vi "Count Update.vi"(8 "error in":errorcluster, 11 "OutputClusterIn":T1={"Acknowledgement"={"Enqueuer"=refnum, "VIReference"=refnum, "VIName"=""}, "AllPartInfo"=[{"PartName"="", "NumberOfRacks"=0, "MeasurementIDsArray"=[], "MeasurementNamesArray"=[], "SpecValuesArray"=[]}], "PartInfo"={"PartName"="", "TotalCount"=0, "ReelCount"=0, "NumberOfRacks"=0, "MeasurementIDsArray"=[], "MeasurementNamesArray"=[], "SpecValuesArray"=[]}, "Result Cluster"={"Measurement Names Array"=[], "Pass-Fail Array"=[], "Measurement Values Array "=[], "Roi for overlay (Arrows) Array"=[], "Algo Type Array"=[], "Image Array"=[], "Clamp operations"=enum."Average Clamp", "  Search Direction "=[], "Images_Array_in"=[], "ResultPF"=FALSE, "Total Cluster Values"={"Total Fail"=0, "Total Pass"=0, "Total Count"=0}, "Reel Counter Cluster"={"Reel Fail"=0, "Reel Pass"=0, "Reel Count"=0}, "Tolerance  Array"=[], "Array of Cam Spec Control Bool"=[], "Control Pass Fail Array"=[], "Specification Pass Fail Array"=[], "Overlay Arrow Lines"=[], "Camera ID"=[], "Trigger count"=0, "Specification fail?"=FALSE}, "ErrorMessage"=""}) -> (0 "error out":errorcluster, 3 "OutputClusterOut":T1={"Acknowledgement"={"Enqueuer"=refnum, "VIReference"=refnum, "VIName"=""}, "AllPartInfo"=[{"PartName"="", "NumberOfRacks"=0, "MeasurementIDsArray"=[], "MeasurementNamesArray"=[], "SpecValuesArray"=[]}], "PartInfo"={"PartName"="", "TotalCount"=0, "ReelCount"=0, "NumberOfRacks"=0, "MeasurementIDsArray"=[], "MeasurementNamesArray"=[], "SpecValuesArray"=[]}, "Result Cluster"={"Measurement Names Array"=[], "Pass-Fail Array"=[], "Measurement Values Array "=[], "Roi for overlay (Arrows) Array"=[], "Algo Type Array"=[], "Image Array"=[], "Clamp operations"=enum."Average Clamp", "  Search Direction "=[], "Images_Array_in"=[], "ResultPF"=FALSE, "Total Cluster Values"={"Total Fail"=0, "Total Pass"=0, "Total Count"=0}, "Reel Counter Cluster"={"Reel Fail"=0, "Reel Pass"=0, "Reel Count"=0}, "Tolerance  Array"=[], "Array of Cam Spec Control Bool"=[], "Control Pass Fail Array"=[], "Specification Pass Fail Array"=[], "Overlay Arrow Lines"=[], "Camera ID"=[], "Trigger count"=0, "Specification fail?"=FALSE}, "ErrorMessage"=""})   [LabVIEW 2019, in "Algorithm.lvclass"]
uses:
  FrameworkOverrides/Algorithm.lvclass
  Controls/OutputCluster.ctl
  Common/Controls/AllPartInfo.ctl
  Common/Controls/Acknowledgement.ctl
  <vilib>/ActorFramework/Message Enqueuer/Message Enqueuer.lvclass
  Controls/Result Cluster.ctl
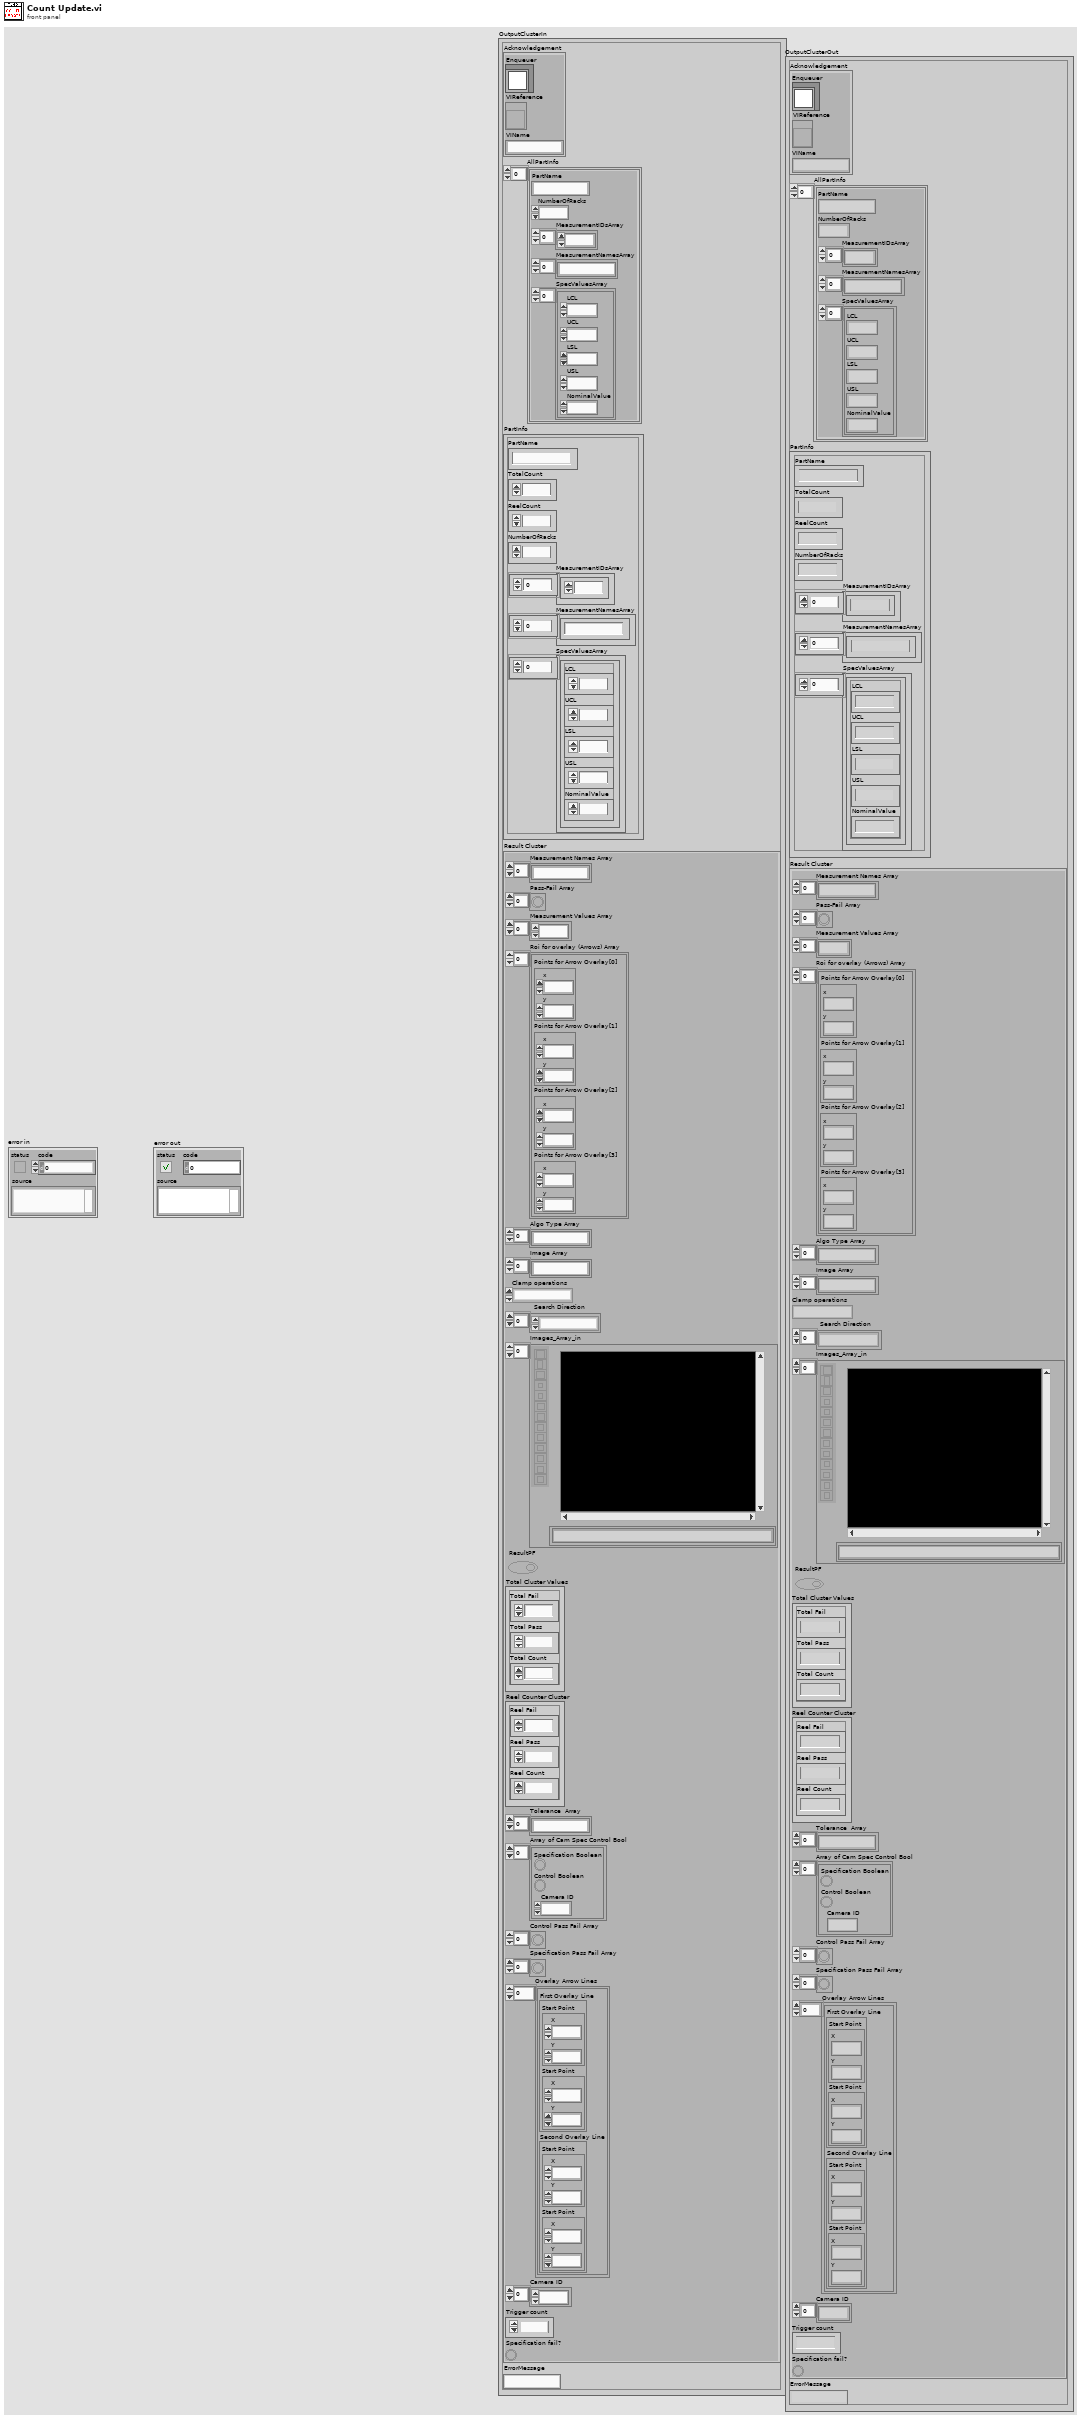
[diagram p1: front panel]
types:
  T1 = typedef "Algorithm.lvclass/OutputCluster.ctl" = cluster{"Acknowledgement":T2, "AllPartInfo":T3, "PartInfo":cluster{"PartName":string, "TotalCount":u64, "ReelCount":u64, "NumberOfRacks":u8, "MeasurementIDsArray":u16[], "MeasurementNamesArray":string[], "SpecValuesArray":cluster{"LCL":dbl, "UCL":dbl, "LSL":dbl, "USL":dbl, "NominalValue":dbl}[]}, "Result Cluster":T4, "ErrorMessage":string}
  T2 = typedef "Acknowledgement.ctl" = cluster{"Enqueuer":refnum<class "Message Enqueuer.lvclass">, "VIReference":refnum<vi>, "VIName":string}
  T3 = typedef "AllPartInfo.ctl" = cluster{"PartName":string, "NumberOfRacks":u8, "MeasurementIDsArray":u16[], "MeasurementNamesArray":string[], "SpecValuesArray":cluster{"LCL":dbl, "UCL":dbl, "LSL":dbl, "USL":dbl, "NominalValue":dbl}[]}[]
  T4 = typedef "Algorithm.lvclass/Result Cluster.ctl" = cluster{"Measurement Names Array":string[], "Pass-Fail Array":bool[], "Measurement Values Array ":dbl[], "Roi for overlay (Arrows) Array":cluster{"Points for Arrow Overlay[0]":cluster{"x":dbl, "y":dbl}, "Points for Arrow Overlay[1]":cluster{"x":dbl, "y":dbl}, "Points for Arrow Overlay[2]":cluster{"x":dbl, "y":dbl}, "Points for Arrow Overlay[3]":cluster{"x":dbl, "y":dbl}}[], "Algo Type Array":string[], "Image Array":string[], "Clamp operations":enum16{"Min Clamp", "Max Clamp", "Average Clamp"}, "  Search Direction ":enum16{"Left to Right", "Right to Left", "Top to Bottom", "Bottom to Top"}[], "Images_Array_in":T5[], "ResultPF":bool, "Total Cluster Values":cluster{"Total Fail":u64, "Total Pass":u64, "Total Count":u64}, "Reel Counter Cluster":cluster{"Reel Fail":u64, "Reel Pass":u64, "Reel Count":u64}, "Tolerance  Array":string[], "Array of Cam Spec Control Bool":cluster{"Specification Boolean":bool, "Control Boolean":bool, "Camera ID":i8}[], "Control Pass Fail Array":bool[], "Specification Pass Fail Array":bool[], "Overlay Arrow Lines":cluster{"First Overlay Line ":cluster{"Start Point":cluster{"X":sgl, "Y":sgl}, "Start Point":cluster{"X":sgl, "Y":sgl}}, "Second Overlay Line ":cluster{"Start Point":cluster{"X":sgl, "Y":sgl}, "Start Point":cluster{"X":sgl, "Y":sgl}}}[], "Camera ID":i8[], "Trigger count":i32, "Specification fail?":bool}
  T5 = typedef "IMAQ Image.ctl" = refnum<image>
  T6 = cluster{"Total Fail":u64, "Total Pass":u64, "Total Count":u64}
  T7 = cluster{"Reel Fail":u64, "Reel Pass":u64, "Reel Count":u64}
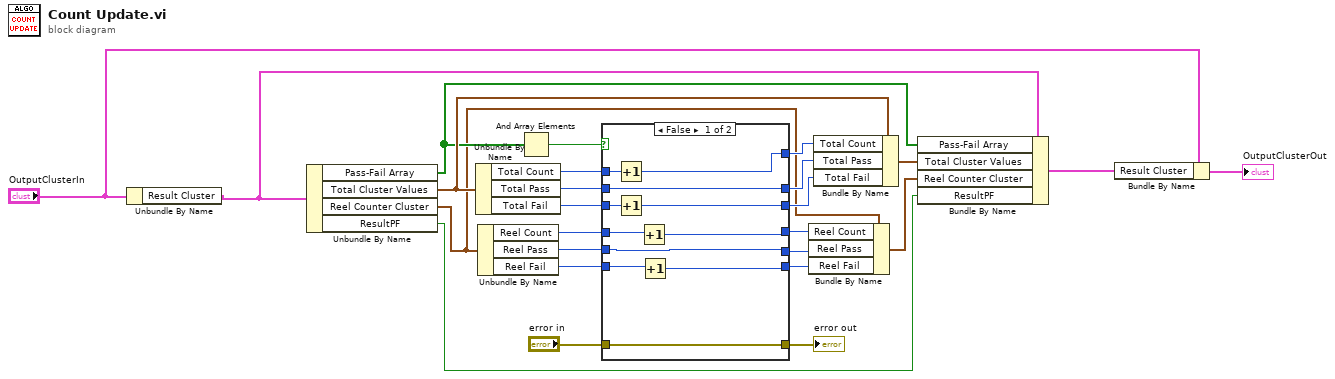
[diagram p0: block diagram]
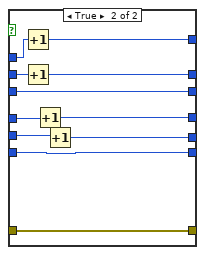
[diagram p2: hidden frame]
diagram:
  n1 = Unbundle By Name("OutputClusterIn") -> ("Result Cluster"=w4:T4)
  n2 = Unbundle By Name(w4) -> ("Pass-Fail Array"=w17:bool[], "Total Cluster Values"=w18:T6, "Reel Counter Cluster"=w6:T7, "ResultPF"=w15:bool)
  n3 = Unbundle By Name(w18) -> ("Total Count"=w20:u64, "Total Pass"=w22:u64, "Total Fail"=w23:u64)
  n4 = Unbundle By Name(w6) -> ("Reel Count"=w12:u64, "Reel Pass"=w11:u64, "Reel Fail"=w10:u64)
  n5 = And Array Elements(Boolean array=w17) -> (logical AND=w21:bool)
  n6 = case shown="False" w21 {
    tunnel: w22 -> [w36 w47]
    tunnel: w23 -> [w35 w46]
    tunnel: [w36 w45] -> w24
    tunnel: [w34 w46] -> w25
    tunnel: w20 -> [w33 w44]
    tunnel: [w32 w43] -> w19
    tunnel: [w31 w42] -> w14
    tunnel: "error in" -> [w31 w42]
    tunnel: w12 -> [w28 w41]
    tunnel: w11 -> [w26 w39]
    tunnel: w10 -> [w30 w37]
    tunnel: [w27 w40] -> w9
    tunnel: [w26 w38] -> w8
    tunnel: [w29 w37] -> w7
    frame False {
      n7 = Increment(x=w33) -> (x+1=w32:u64)
      n8 = Increment(x=w35) -> (x+1=w34:u64)
      n9 = Increment(x=w28) -> (x+1=w27:u64)
      n10 = Increment(x=w30) -> (x+1=w29:u64)
    }
    frame True {
      n11 = Increment(x=w44) -> (x+1=w43:u64)
      n12 = Increment(x=w47) -> (x+1=w45:u64)
      n13 = Increment(x=w41) -> (x+1=w40:u64)
      n14 = Increment(x=w39) -> (x+1=w38:u64)
    }
  }
  "error out" <- w14
  n15 = Bundle By Name(cluster=w6, "Reel Count"=w9, "Reel Pass"=w8, "Reel Fail"=w7) -> (w5:T7)
  n16 = Bundle By Name(cluster=w18, "Total Count"=w19, "Total Pass"=w24, "Total Fail"=w25) -> (w16:T6)
  n17 = Bundle By Name(cluster=w4, "Pass-Fail Array"=w17, "Total Cluster Values"=w16, "Reel Counter Cluster"=w5, "ResultPF"=w15) -> (w2:T4)
  n18 = Bundle By Name(cluster="OutputClusterIn", "Result Cluster"=w2) -> (→"OutputClusterOut":T1)
